vi "PQputCopyEnd.vi"(8 "error in (no error)":errorcluster, 10 "errormsg":string) -> (0 "error out":errorcluster, 2 "PQputCopyEnd":i32)   [LabVIEW 2019, in "libpqlv.lvlib"]
uses:
  libpqlv.lvlib
  libpq.dll
panel:
  in  "conn":u32
  out "conn_out":u32
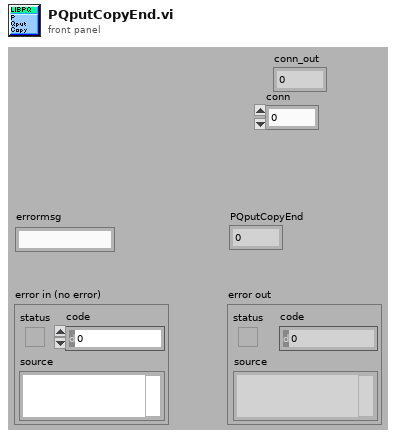
[diagram p1: front panel]
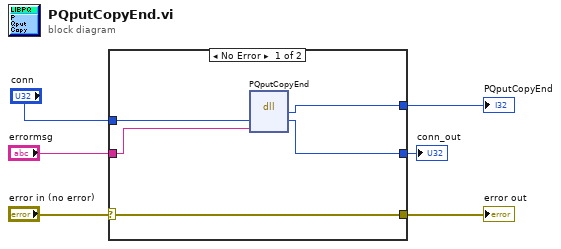
[diagram p0: block diagram]
diagram:
  n1 = case shown="No Error" "error in (no error)" {
    selector: "error in (no error)" -> [w11 w13]
    tunnel: [w11 w13] -> w5
    tunnel: [w10 _] -> w4
    tunnel: [w9 w12] -> w2
    tunnel: "errormsg" -> [w8 _]
    tunnel: "conn" -> [w7 w12]
    frame No Error {
      n2 = dll-call lib="libpq.*" fn="PQputCopyEnd"("conn"=w7, "errormsg"=w8) -> ("PutCopyEnd"=w10:i32, "conn"=w9:u32)  [unwired: 4 in, 2 out]
    }
    frame Error {
    }
  }
  "PQputCopyEnd" <- w4
  "error out" <- w5
  "conn_out" <- w2
